vi "TestPowermeter.vi"() -> ()   [LabVIEW 2018]
uses:
  <instrlib>/Classes/Powermeter/Thorlabs_PM100D/Thorlabs_PM100D.lvclass
panel:
  out "x/y":dbl
  out "mean":dbl format="%0.2f"
  out "Array":dbl[](array[numeric])
  out "Wavelength (m) 3":dbl
  out "Wavelength (m) 2":dbl
  in  "Wavelength (m)":dbl
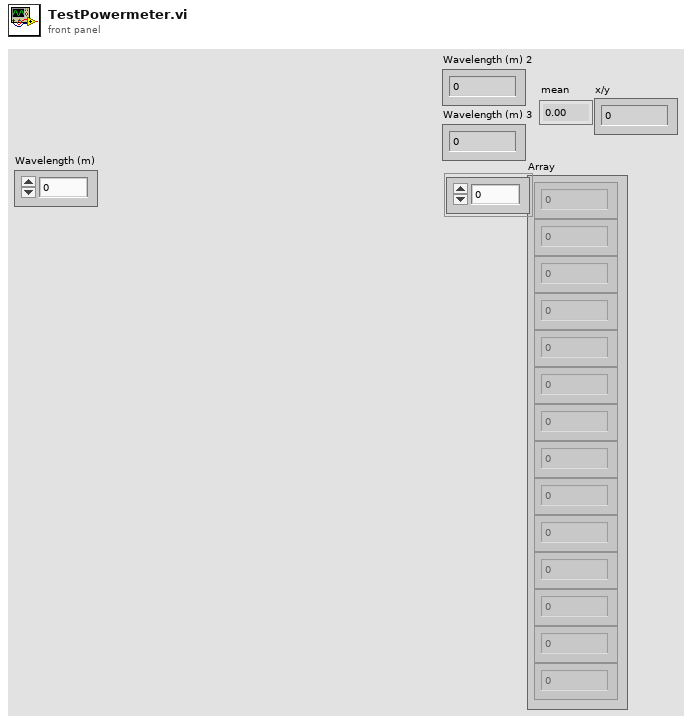
[diagram p1: front panel]
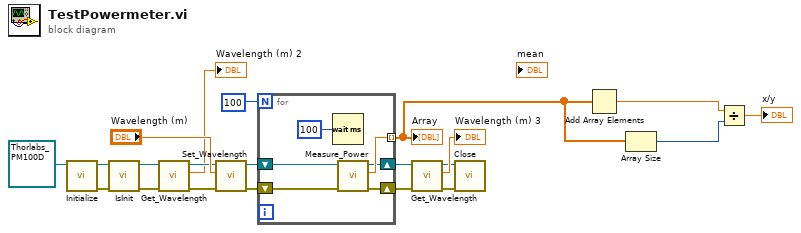
[diagram p0: block diagram]
diagram:
  n1 = call-dynamic "Initialize.vi"("Thorlabs_PM100D in"=refnum<class "Thorlabs_PM100D.lvclass"> refnum ("Thorlabs_PM100D.lvclass")) -> ("error out"=w17:errorcluster, "Thorlabs_PM100D out"=w19:refnum<class "Thorlabs_PM100D.lvclass">)  [unwired: 9 in]
  n2 = call-dynamic "IsInit.vi"("error in (no error)"=w17, "Thorlabs_PM100D in"=w19) -> ("error out"=w13:errorcluster, "Thorlabs_PM100D out"=w14:refnum<class "Thorlabs_PM100D.lvclass">)  [unwired: 7 in, 1 out]
  n3 = call-dynamic "Get_Wavelength.vi"("error in (no error)"=w13, "Thorlabs_PM100D in"=w14) -> ("error out"=w11:errorcluster, "Wavelength (m)"=→"Wavelength (m) 2":dbl, "Thorlabs_PM100D out"=w12:refnum<class "Thorlabs_PM100D.lvclass">)  [unwired: 7 in]
  n4 = call-dynamic "Set_Wavelength.vi"("error in (no error)"=w11, "Wavelength (m)"="Wavelength (m)", "Thorlabs_PM100D in"=w12) -> ("error out"=w20:errorcluster, "Thorlabs_PM100D out"=w21:refnum<class "Thorlabs_PM100D.lvclass">)  [unwired: 7 in]
  n5 = for {
    N: 100 -> [_]
    tunnel: [w26] -> w4 mode=indexing
    shift-right: [w24] -> w9
    shift-left: w21 -> [w25]
    shift-right: [w23] -> w10
    shift-left: w20 -> [w22]
    n6 = Wait (ms)(milliseconds to wait=u32 100) -> ()  [unwired: 1 out]
    n7 = call-dynamic "Measure_Power.vi"("error in (no error)"=w22, "Thorlabs_PM100D in"=w25) -> ("error out"=w23:errorcluster, "Power (W)"=w26:dbl, "Thorlabs_PM100D out"=w24:refnum<class "Thorlabs_PM100D.lvclass">)  [unwired: 7 in]
  }
  "Array" <- w4
  n8 = call-dynamic "Get_Wavelength.vi"("error in (no error)"=w10, "Thorlabs_PM100D in"=w9) -> ("error out"=w5:errorcluster, "Wavelength (m)"=→"Wavelength (m) 3":dbl, "Thorlabs_PM100D out"=w6:refnum<class "Thorlabs_PM100D.lvclass">)  [unwired: 7 in]
  n9 = call-dynamic "Close.vi"("error in (no error)"=w5, "Thorlabs_PM100D in"=w6) -> ()  [unwired: 8 in, 2 out]
  n10 = Add Array Elements(numeric array=w4) -> (sum=w3:dbl)
  n11 = Array Size(array=w4) -> (size(s)=w2:i32)
  n12 = Divide(x=w3, y=w2) -> (x/y=→"x/y":dbl)
